vi "Draw_polygon_exercise_ms2.vi"() -> ()   [LabVIEW 2016]
uses:
  Classes/Controller/Motion/A3200 Folder/A3200.lvclass
panel:
  in  "Speed":dbl=20.0
  in  "array/Axis":bool
  in  "initial_angle":dbl
  in  "d":dbl=20.0
  in  "Numeric":i32=2
  in  "P_num":i32=6
  in  "r":dbl=100.0
  in  "c_y":dbl=500.0
  in  "c_x":dbl=500.0
  out "Array 3":dbl[](array[numeric])
  out "Array 2":dbl[][](array[numeric])
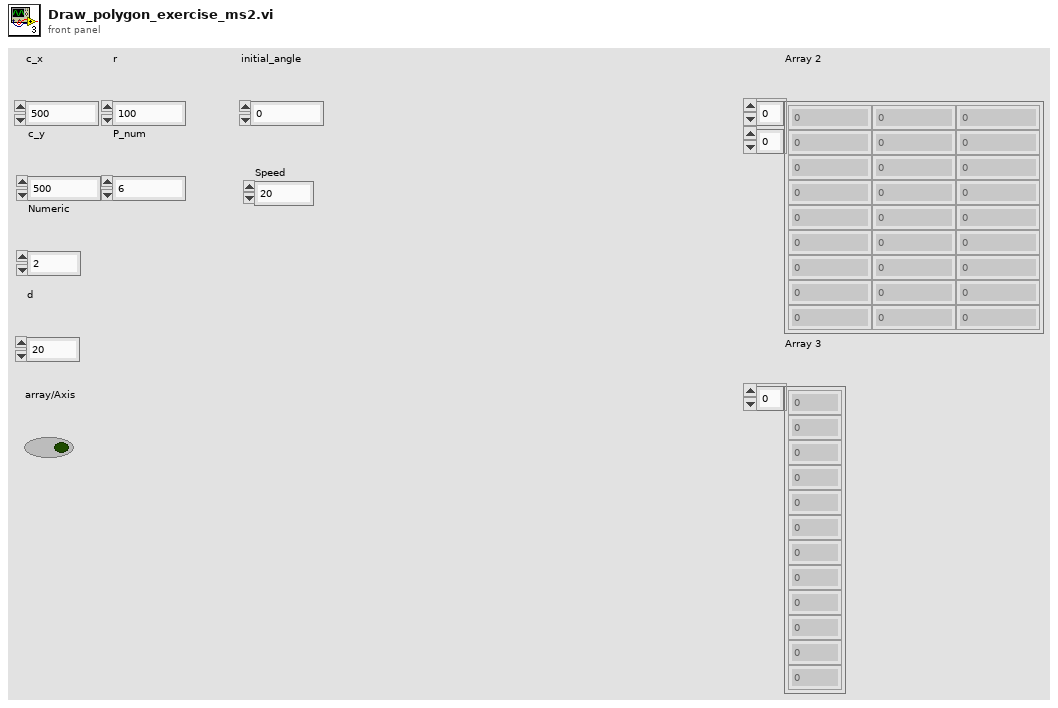
[diagram p1: front panel]
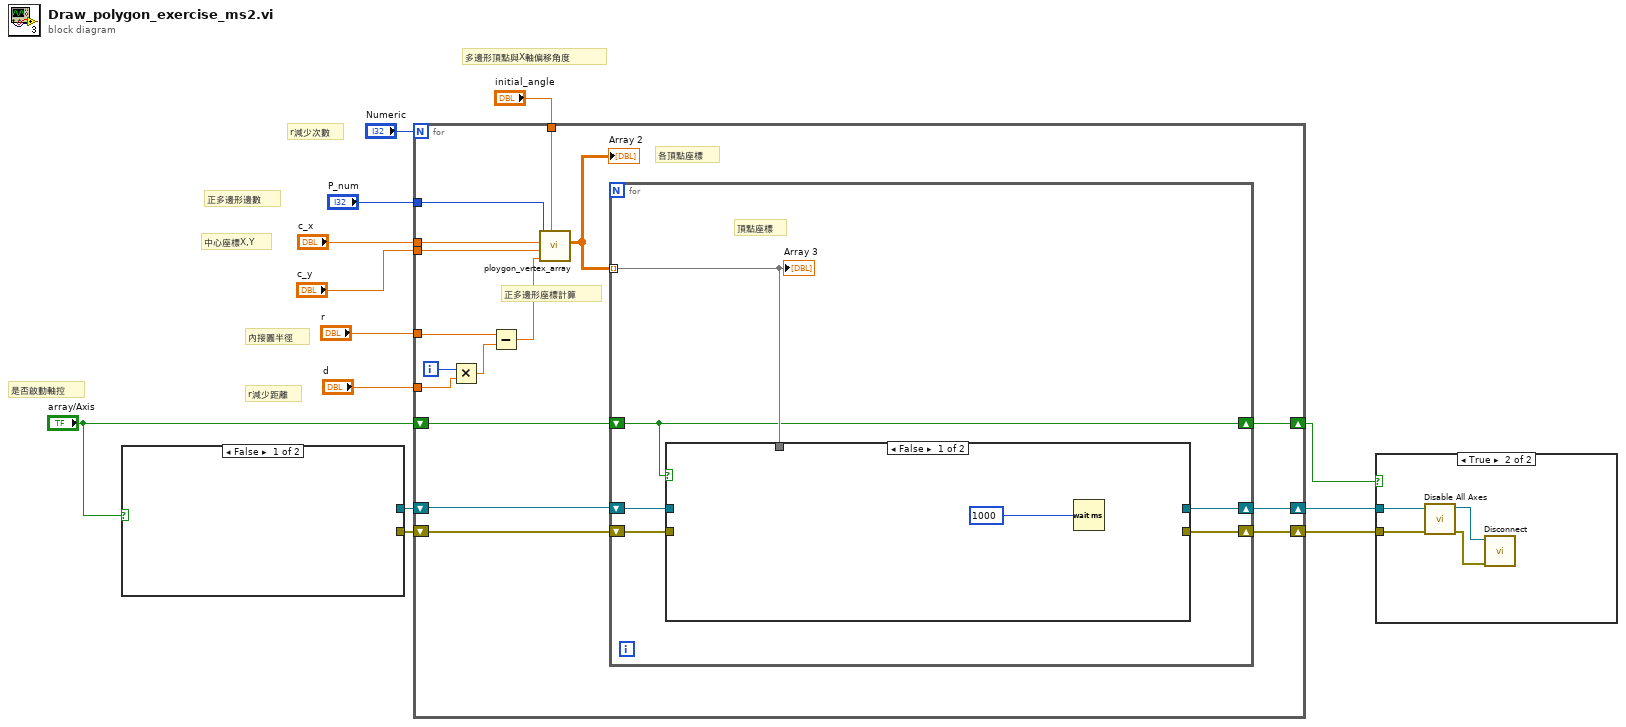
[diagram p0: block diagram]
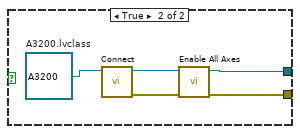
[diagram p3: hidden frame]
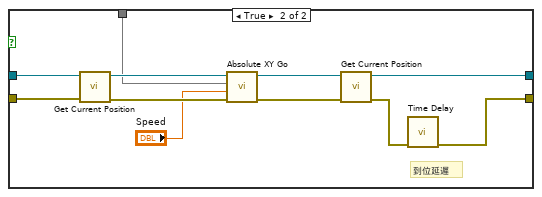
[diagram p4: hidden frame]
diagram:
  # "是否啟動軸控"
  # "多邊形頂點與X軸偏移角度"
  # "r減少次數"
  # "正多邊形邊數"
  # "中心座標X,Y"
  # "內接圓半徑"
  # "r減少距離"
  n1 = case shown="False" "array/Axis" {
    tunnel: [_ w15] -> w2
    tunnel: [_ w14] -> w1
    frame False {
    }
    frame True {
      w18 = refnum<class "A3200.lvclass"> refnum  # A3200.lvclass
      n2 = call-dynamic "Connect.vi"("Gantry in"=w18) -> ("error out"=w16:errorcluster, "Gantry out"=w17:refnum<class "A3200.lvclass">)  [unwired: 9 in]
      n3 = call-dynamic "Enable All Axes.vi"("error in (no error)"=w16, "A3200 in"=w17) -> ("error out"=w15:errorcluster, "A3200 out"=w14:refnum<class "A3200.lvclass">)  [unwired: 8 in]
    }
  }
  n4 = for {
    N: "Numeric" -> [_]
    tunnel: "c_x" -> [w33]
    tunnel: "c_y" -> [w32]
    tunnel: "r" -> [w28]
    tunnel: "P_num" -> [w31]
    tunnel: "initial_angle" -> [w26]
    tunnel: "d" -> [w25]
    shift-right: [w23] -> w6
    shift-left: w1 -> [w24]
    shift-right: [w22] -> w5
    shift-left: w2 -> [w21]
    shift-right: [w19] -> w3
    shift-left: "array/Axis" -> [w20]
    i -> [w30]
    # "正多邊形座標計算"
    # "各頂點座標"
    n5 = Multiply(x=w30, y=w25) -> (x*y=w29:dbl)
    n6 = Subtract(x=w28, y=w29) -> (x-y=w27:dbl)
    n7 = call "ploygon_vertex_array.vi"("initial_angle"=w26, "r"=w27, "c_y"=w32, "c_x"=w33, "P_num"=w31) -> ("Array 2"=w34:dbl[][])  [unwired: 6 in]
    "Array 2" <- w34
    n8 = for {
      tunnel: w34 -> [w36] mode=indexing
      shift-right: [w40] -> w23
      shift-left: w24 -> [w38]
      shift-right: [w39] -> w22
      shift-left: w21 -> [w37]
      shift-right: [w35] -> w19
      shift-left: w20 -> [w35]
      # "頂點座標"
      n9 = case shown="False" w35 {
        tunnel: [_ w48] -> w40
        tunnel: [_ w50] -> w39
        tunnel: w38 -> [_ w47]
        tunnel: w37 -> [_ w45]
        tunnel: w36 -> [_ w43]
        frame False {
          n10 = Wait (ms)(milliseconds to wait=u32 1000) -> ()  [unwired: 1 out]
        }
        frame True {
          # "到位延遲"
          n11 = call-dynamic "Get Current Position.vi"("error in (no error)"=w45, "Gantry in"=w47) -> ("error out"=w44:errorcluster, "Gantry out"=w46:refnum<class "A3200.lvclass">)  [unwired: 7 in, 1 out]
          n12 = call-dynamic "Absolute XY Go.vi"("error in (no error)"=w44, "Speed"="Speed", "XY"=w43, "Gantry in"=w46) -> ("error out"=w52:errorcluster, "Gantry out"=w49:refnum<class "A3200.lvclass">)  [unwired: 6 in]
          n13 = call-dynamic "Get Current Position.vi"("error in (no error)"=w52, "Gantry in"=w49) -> ("error out"=w51:errorcluster, "Gantry out"=w48:refnum<class "A3200.lvclass">)  [unwired: 7 in, 1 out]
          n14 = call "Time Delay"("error in (no error)"=w51) -> ("error out"=w50:errorcluster)  [unwired: 10 in]
        }
      }
      "Array 3" <- w36
    }
  }
  n15 = case shown="True" w3 {
    tunnel: w6 -> [_ w56]
    tunnel: w5 -> [_ w53]
    frame False {
    }
    frame True {
      n16 = call-dynamic "Disable All Axes.vi"("error in (no error)"=w53, "Gantry in"=w56) -> ("error out"=w54:errorcluster, "Gantry out"=w55:refnum<class "A3200.lvclass">)  [unwired: 8 in]
      n17 = call-dynamic "Disconnect.vi"("error in (no error)"=w54, "Gantry in"=w55) -> ()  [unwired: 8 in, 1 out]
    }
  }
